vi "Read configuration.vi"(8 "error in (no error)":errorcluster, 11 "Device Channel in":refnum<class "Synchronization Channel.lvclass">) -> (0 "error out":errorcluster, 2 "configuration":refnum<class "CEF_serializable configuration.lvclass">, 3 "Device Channel out":refnum<class "Synchronization Channel.lvclass">)   [LabVIEW 2025, in "Synchronization.lvlib" / "Synchronization Channel.lvclass"]
uses:
  Synchronization Channel.lvclass
  Users/Public/Documents/Sandia National Labs/TSS Plugin/CEF.lvlibp/serializable configuration/CEF_serializable configuration.lvclass
  Synchronization Channel.lvclass/Synchronization Channel.ctl
  Synchronization Channel configuration/Synchronization Channel configuration.lvclass
  C:/Users/Public/Documents/Sandia National Labs/TSS Plugin/CEF.lvlibp/serializable configuration/CEF_serializable configuration.lvclass
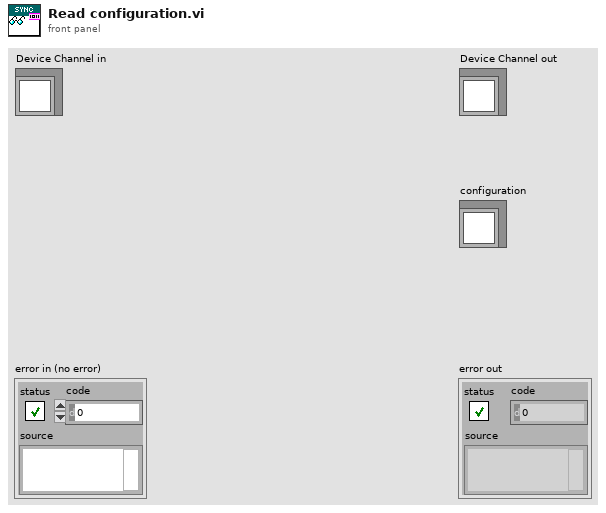
[diagram p1: front panel]
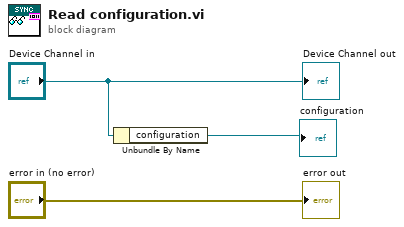
[diagram p0: block diagram]
diagram:
  n1 = Unbundle By Name("Device Channel in") -> ("configuration"=→"configuration":refnum<class "Synchronization Channel configuration.lvclass">)
  "error out" <- "error in (no error)"
  "Device Channel out" <- "Device Channel in"
